vi "LVClass_CorrectionDataManager GetActuatorPrefs.vi"(0 "CorrectionDataManager in":refnum<class "CorrectionDataManager.lvclass">, 5 "N° actuator":i32, 11 "error in (no error)":errorcluster) -> (4 "CorrectionDataManager out":refnum<class "CorrectionDataManager.lvclass">, 6 "Actuator state":T1, 15 "error out":errorcluster)   [LabVIEW 2020, in "CorrectionDataManager.lvclass"]
uses:
  CorrectionDataManager.lvclass
  Wavefront Corrector states - ONE.ctl
  CorrectionDataManager.lvclass/CorrectionDataManager.ctl
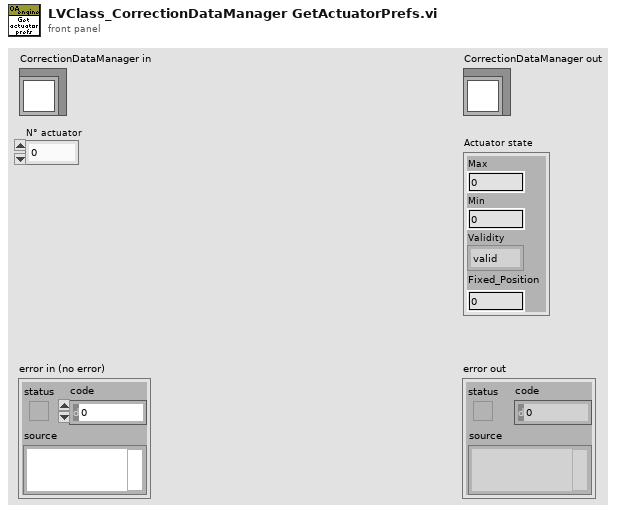
[diagram p1: front panel]
types:
  T1 = typedef "Wavefront Corrector states - ONE.ctl" = cluster{"Max":sgl, "Min":sgl, "Validity":enum16{"valid", "fixed", "invalid"}, "Fixed_Position":sgl}
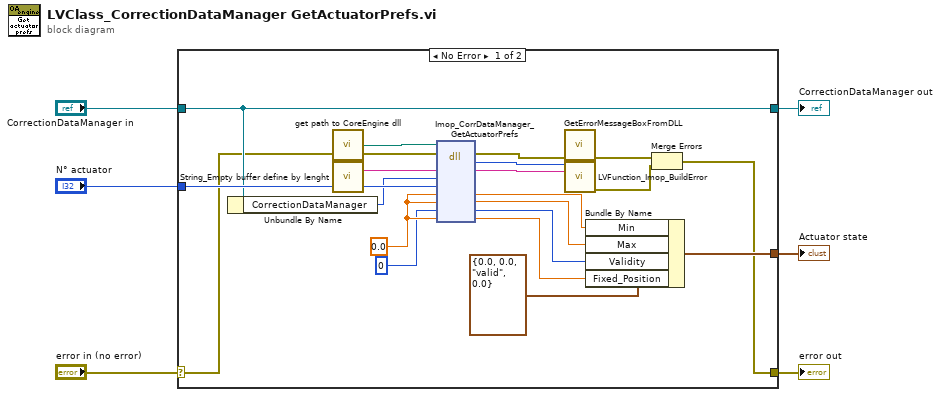
[diagram p0: block diagram]
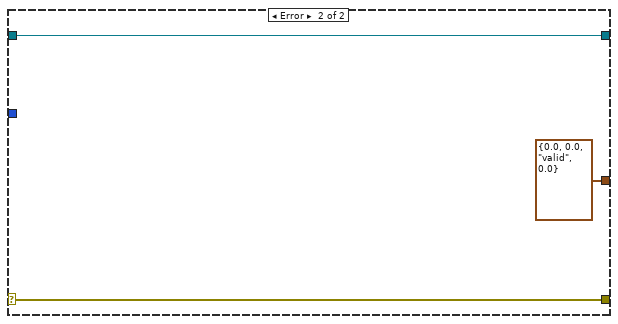
[diagram p2: hidden frame]
diagram:
  n1 = case shown="No Error" "error in (no error)" {
    selector: "error in (no error)" -> [w8 w29]
    tunnel: [w7 w29] -> w5
    tunnel: [w18 w28] -> w3
    tunnel: "CorrectionDataManager in" -> [w18 w28]
    tunnel: "N° actuator" -> [w19 _]
    tunnel: [w9 T1 {"Max"=0.0, "Min"=0.0, "Validity"=enum."valid", "Fixed_Position"=0.0} ("Actuator state")] -> w1
    frame No Error {
      w16 = 0.0
      n2 = Unbundle By Name(w18) -> ("CorrectionDataManager"=w17:i32)
      n3 = call "get path to CoreEngine dll.vi"() -> ("path to c_interface_vc100.dll"=w24:path)  [unwired: 12 in, 3 out]
      n4 = call "String_Empty buffer define by lenght.vi"() -> ("Empty buffer"=w23:string)  [unwired: 1 in]
      n5 = dll-call lib="D:/FLE/0.Code/CoreEngine4_Suite/LV2011_interface/DLLs/c_interface_vc100.dll" fn="Imop_CorrDataManager_GetActuatorPrefs"(path in=w24, error in=w8, "Message"=w23, "CorrectionDataManager"=w17, "Actuator index"=w19, "Min"=w16, "Max"=w16, "Validity"=0, "Fixed position"=w16) -> (error out=w22:errorcluster, "return type"=w21:i32, "Message"=w20:string, "Min"=w13:sgl, "Max"=w12:sgl, "Validity"=w11:i32, "Fixed position"=w10:sgl)  [unwired: 3 in, 1 out]
      n6 = call "GetErrorMessageBoxFromDLL.vi"("error IN"=w22) -> ("error OUT"=w26:errorcluster)  [unwired: 10 in]
      n7 = call "LVFunction_Imop_BuildError.vi"("code"=w21, "String to Prepend to source (\"\")"=w20) -> ("error out"=w25:errorcluster)  [unwired: 13 in]
      n8 = Bundle By Name(cluster=T1 {"Max"=0.0, "Min"=0.0, "Validity"=enum."valid", "Fixed_Position"=0.0} ("Actuator state"), "Min"=w13, "Max"=w12, "Validity"=w11, "Fixed_Position"=w10) -> (w9:T1)
      n9 = Merge Errors(w26, w25) -> (w7:errorcluster)
    }
    frame Error {
    }
  }
  "error out" <- w5
  "CorrectionDataManager out" <- w3
  "Actuator state" <- w1
